vi "Cache.Global.vi"() -> ()   [LabVIEW 2016]
uses:
  Cache.Data.Sets.ctl
panel:
  in  "Logger.Sets":T1
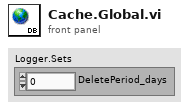
[diagram p1: front panel]
types:
  T1 = typedef "Cache.Data.Sets.ctl" = cluster{"DeletePeriod_days":dbl}
diagram:
